vi "Close.vi"(8 "error in (no error)":errorcluster, 11 "bt_System in":refnum<class "bt_System.lvclass">) -> (0 "error out":errorcluster, 3 "bt_System out":refnum<class "bt_System.lvclass">)   [LabVIEW 2021, in "BT.lvlib" / "bt_System.lvclass"]
uses:
  bt_System.lvclass
  bt_System.lvclass/bt_System.ctl
  Support/Nodes/abs_Node/bt_Node.lvclass
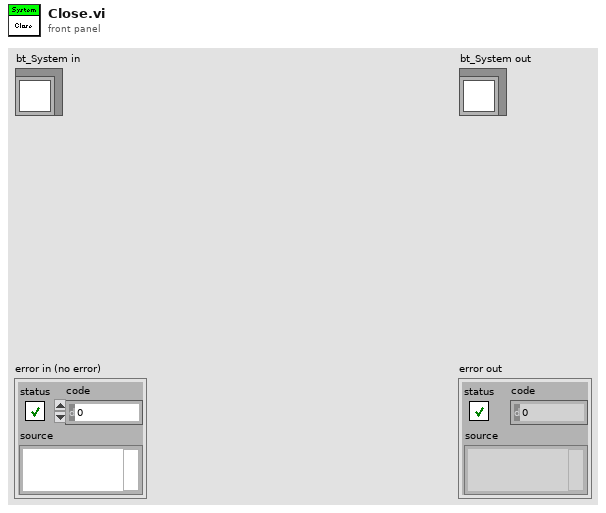
[diagram p1: front panel]
types:
  T1 = typedef "Rendezvous RefNum" = refnum<k1>
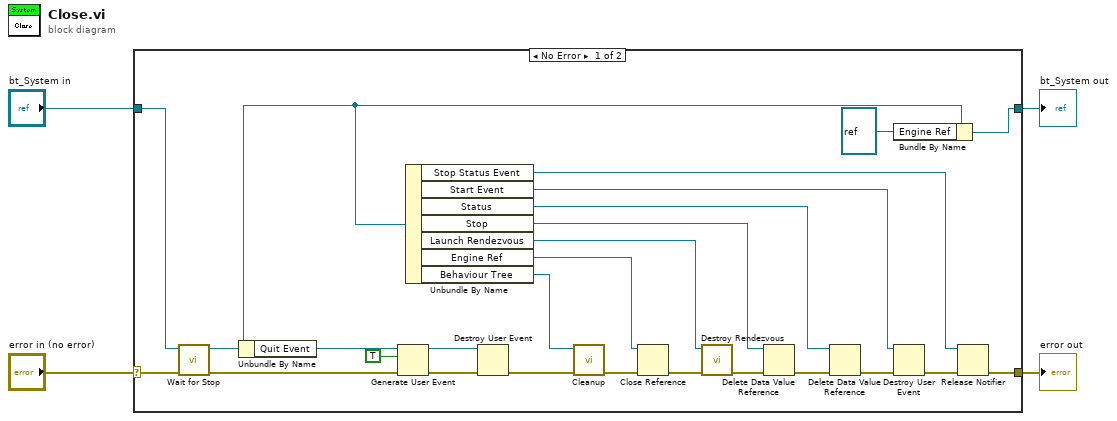
[diagram p0: block diagram]
diagram:
  n1 = case shown="No Error" "error in (no error)" {
    selector: "error in (no error)" -> [w11 w31]
    tunnel: [w17 w31] -> w3
    tunnel: [w28 w30] -> w1
    tunnel: "bt_System in" -> [w10 w30]
    frame No Error {
      n2 = call "Wait for Stop.vi"("error in (no error)"=w11, "bt_System in"=w10) -> ("error"=w8:errorcluster, "bt_System out"=w9:refnum<class "bt_System.lvclass">)  [unwired: 6 in, 2 out]
      n3 = Unbundle By Name(w9) -> ("Quit Event"=w13:refnum<user-event>)
      n4 = Generate User Event(user event=w13, event data cluster=TRUE ("event data"), error in=w8) -> (user event out=w7:refnum<user-event>, error out=w6:errorcluster)  [unwired: 1 in]
      n5 = Unbundle By Name(w9) -> ("Stop Status Event"=w15:refnum<notifier>, "Start Event"=w16:refnum<user-event>, "Status"=w19:refnum<data-value>, "Stop"=w21:refnum<data-value>, "Launch Rendezvous"=w25:T1, "Engine Ref"=w29:refnum<vi>, "Behaviour Tree"=w24:refnum<class "bt_Node.lvclass">)
      n6 = Destroy User Event(user event=w7, error in=w6) -> (error out=w5:errorcluster)
      n7 = call-dynamic "Cleanup.vi"("error in (no error)"=w5, "Node in"=w24) -> ("error out"=w23:errorcluster)  [unwired: 8 in, 1 out]
      n8 = Close Reference(reference=w29, error in (no error)=w23) -> (error out=w26:errorcluster)
      n9 = call <vilib>:"Destroy Rendezvous.vi"("error in (no error)"=w26, "rendezvous"=w25) -> ("error out"=w22:errorcluster)  [unwired: 4 in, 1 out]
      n10 = Delete Data Value Reference(data value reference=w21, error in=w22) -> (error out=w20:errorcluster)  [unwired: 1 out]
      n11 = Delete Data Value Reference(data value reference=w19, error in=w20) -> (error out=w18:errorcluster)  [unwired: 1 out]
      n12 = Bundle By Name(cluster=w9, "Engine Ref"=refnum<vi> refnum) -> (w28:refnum<class "bt_System.lvclass">)
      n13 = Destroy User Event(user event=w16, error in=w18) -> (error out=w14:errorcluster)
      n14 = Release Notifier(notifier=w15, error in (no error)=w14) -> (error out=w17:errorcluster)  [unwired: 1 in, 2 out]
    }
    frame Error {
    }
  }
  "error out" <- w3
  "bt_System out" <- w1
